vi "create GWS lvhttp config.vi"(4 "error in (no error)":errorcluster) -> (0 "error out":errorcluster)   [LabVIEW 2011]
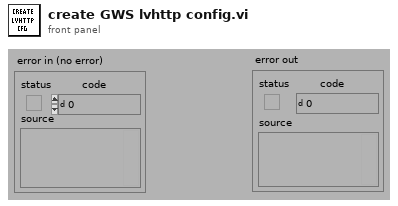
[diagram p1: front panel]
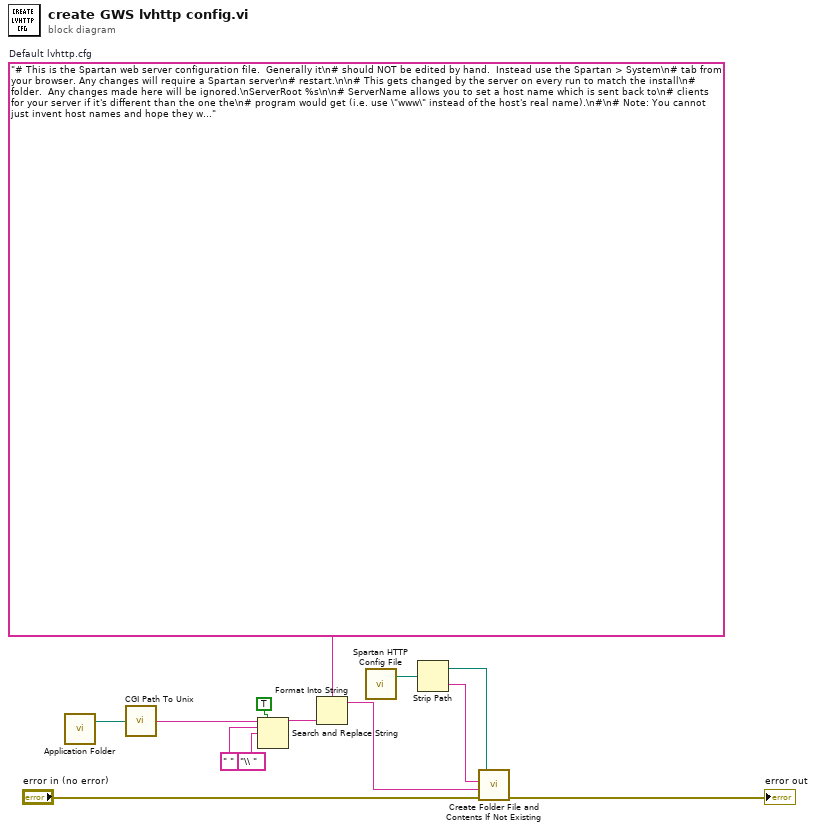
[diagram p0: block diagram]
diagram:
  w7 = "# This is the Spartan web server configuration file.  Generally it\n# should NOT be edited by hand.  Instead use the Spartan > System\n# tab from your browser. Any changes will require a Spartan server\n# restart.\n\n# This gets changed by the server on every run to match the install\n# folder.  Any changes made here will be ignored.\nServerRoot %s\n\n# ServerName allows you to set a host name which is sent back to\n# clients for your server if it's different than the one the\n# program would get (i.e. use \"www\" instead of the host's real name).\n#\n# Note: You cannot just invent host names and hope they work.\n# The name you define here must be a valid DNS name for your\n# host. If you don't understand this, ask your network\n# administrator.  Format: ServerName new.host.name\nServerName\n\n# ServerAdmin: The email address, where problems with the server should be\n# e-mailed.\nServerAdmin\n\n# ServerSMTP: The email server to be used by Spartan.  Can be IP or DNS\n# name.\nServerSMTP\n\n# Port: The port to which the web server listens for incoming requests.\n# Web servers generally listen to port 80, but any port is valid as long\n# as it's not already in use by another process.\nPort 80\n\n# Determines whether logging, etc. will use DNS format.  If your\n# DNS doesn't resolve, then setting this to on may lead to longer\n# page loads and a slowdown of the system.\nUseDNS off\n\n# Number of connections that may wait for processing.  If MaxPending\n# connections are in the queue, the server will not listen for others\n# until at least one is processed.  A \"server busy\" page will be\n# returned to the requester when the queue is full.\nMaxPending\t100\n\n# Default time (in seconds) that idle CGIs are cached.  This setting\n# controls how long CGI's (really VIT's) remain in server memory after\n# calls.  This is an obsolete setting as of version 3.0, as CGI's are\n# now always single-call (i.e., a new CGI is spawned for every\n# request).\nCGICacheTime\t120\n\n# Set how many connection handlers should run (1-8).  This is the number\n# of incoming request queue handlers that Spartan starts.  For heavy loads\n# this number can be set higher to keep the queue from hitting MaxPending\n# limit too soon.\nStartServers\t4\n\n# Uncomment the following lines to disable logging.  Log files by default\n# will be saved in ServerRoot/logs folder.\n#ErrorLog /dev/null\n#RefererLog /dev/null\n#TransferLog /dev/null\n#AgentLog /dev/null\n\n\n#################################################################\n#\n#  LEGACY SETTINGS BELOW\n#\n#  These settings are held over from the early days when this\n#  was the G Web Server configuration file.  They closely match\n#  settings that were available in Apache at that time, so you\n#  might find information about them by looking at Apache\n#  documentation.  Mostly, though they are not used and are\n#  ignored by Spartan, so they might go away in the future.\n\n# Frequency at which FP image cache is a compacted\nPanelImageCacheCompactTime\t300\n\n# Maximum number of simultaneous server push connections\n# New request will either time out old ones or receive a still image\nServerPushMaxConnections\t40\n\n# Minimum time a server push will be sustained before it may be terminated\n# due to a new request\nServerPushMinTime \t\t240\n\n# Default depth of panel images (1, 4, 8, 24)\nPanelImageDepth\t\t8\n\n# Default quality of panel images (0-100)\nPanelImageQuality\t80\n\n# Default image type of panel images (jpeg)\nPanelImageType\t\tjpeg\n\n# Default refresh rate (in seconds) for animated images\nServerPushRefresh\t\t10\n\n# Default life span (in seconds) of animated images\nServerPushLifeSpan\t\t300\n"  # Default lvhttp.cfg
  n1 = call "Application Folder.vi"() -> ("Application Folder"=w11:path)  [unwired: 3 in]
  n2 = call "CGI Path To Unix.vi"("platform path"=w11) -> ("unix path"=w2:string)  [unwired: 1 in]
  n3 = Search and Replace String(replace all?=TRUE ("replace all? (F)"), input string=w2, search string=" ", replace string="\\ " ("replace string (\"\")")) -> (result string=w1:string)  [unwired: 1 in, 6 out]
  n4 = Format Into String(format string=w7, w1) -> (resulting string=w6:string)  [unwired: 2 in, 1 out]
  n5 = call "Spartan HTTP Config File.vi"() -> ("HTTP Configuration File"=w10:path)  [unwired: 1 out]
  n6 = Strip Path(path=w10) -> (stripped path=w9:path, name=w8:string)
  n7 = call "Create Folder File and Contents If Not Existing.vi"("error in (no error)"="error in (no error)", "File contents to write (\"\")"=w6, "Filename (\"\")"=w8, "File Folder (Empty)"=w9) -> ("error out"=→"error out":errorcluster)  [unwired: 3 out]
